vi "operate.vi"(0 "reference in":refnum<class "File Controller.lvclass">, 5 "error in (no error)":errorcluster) -> (14 "reference out":refnum<class "File Controller.lvclass">, 19 "error out":errorcluster)   [LabVIEW 2015, in "File Controller.lvclass"]
uses:
  File Controller.lvclass
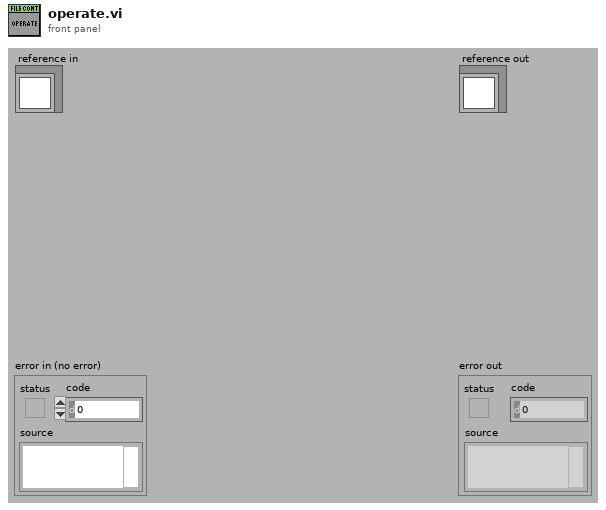
[diagram p1: front panel]
types:
  T1 = typedef "File Controller.lvclass/ObjectAttributesRef.ctl" = refnum<data-value>
  T2 = typedef "File Controller.lvclass/ObjectAttributes.ctl" = cluster{"MyAttribute":dbl, "file_path":path, "file_type":T3, "data":string[][][], "excel_file_ref":refnum<class "excelFile.lvclass">, "sheetName":string[], "subject_refs":refnum<class "subject.lvclass">[], "temp_data":string[][][]}
  T3 = typedef "excelFile.lvclass/fileType.ctl" = enum16{"database", "CosmedTest PFTSUITE", "CosmedTest OMNIA"}
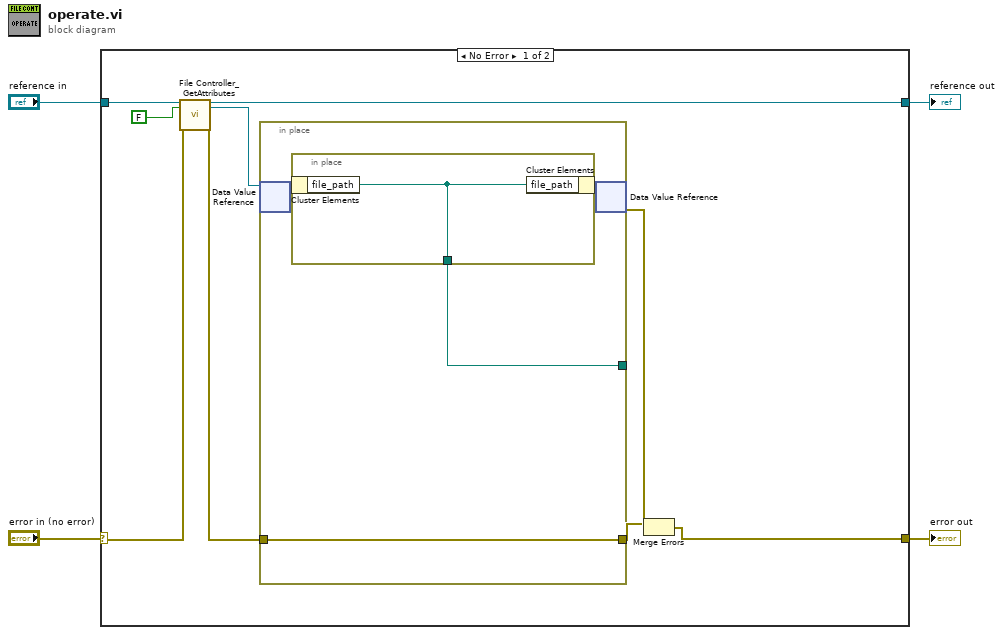
[diagram p0: block diagram]
diagram:
  n1 = case shown="No Error" "error in (no error)" {
    selector: "error in (no error)" -> [w9 w20]
    tunnel: [w5 w20] -> w3
    tunnel: [w7 w19] -> w1
    tunnel: "reference in" -> [w11 w19]
    frame No Error {
      n2 = call "File Controller_GetAttributes.vi"("reference in"=w11, "return data? (T)"=FALSE, "error in (no error)"=w9) -> ("reference out"=w7:refnum<class "File Controller.lvclass">, "attributes ref"=w6:T1, "error out"=w8:errorcluster)  [unwired: 13 in, 1 out]
      n3 = in-place {
        in-place-border: w8 -> [w15]
        in-place-border: [w15] -> w12
        in-place-border: [w14] -> _
        n4 = in-place-dvr #1(w6) -> (w16:T2)  [unwired: 1 out]
        n5 = in-place {
          in-place-border: [w18] -> w14
          n6 = in-place-cluster #2(w16) -> ("file_path"=w18:path)
          n7 = in-place-cluster #2("file_path"=w18) -> (w17:T2)
        }
        n8 = in-place-dvr #1(w17) -> (w13:errorcluster)  [unwired: 1 out]
      }
      n9 = Merge Errors(w12, w13) -> (w5:errorcluster)
    }
    frame Error {
    }
  }
  "error out" <- w3
  "reference out" <- w1
